vi "Read Meta Data (Serial Clst).vi"(8 "error in":errorcluster, 9 "options":T3={"ignore timeout error"=TRUE, "timeout ms (1000)"=1000}, 11 "connection info in":T1) -> (0 "error out":errorcluster, 1 "meta data":T2[](array[typedef]), 3 "connection info out":T1)   [LabVIEW 2013, in "NI STM.lvlib"]
doc: "This VI reads the meta data information from a remote computer. Use this VI to retrieve the variable names and types that a remote computer exports.\n\nThis VI parses the data and returns a cluster containing the meta data information."
uses:
  NI STM.lvlib
  SubVIs/MetaDataElement.ctl
  Serial Read Options.ctl
  Serial Connection Info.ctl
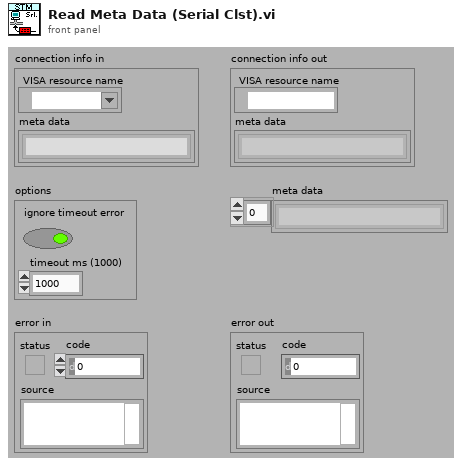
[diagram p1: front panel]
types:
  T1 = typedef "NI STM.lvlib/Serial Connection Info.ctl" = cluster{"VISA resource name":refnum<visa-resource-name>, "meta data":T2[]}
  T2 = typedef "NI STM.lvlib/MetaDataElement.ctl" = string
  T3 = typedef "NI STM.lvlib/Serial Read Options.ctl" = cluster{"ignore timeout error":bool, "timeout ms (1000)":u32}
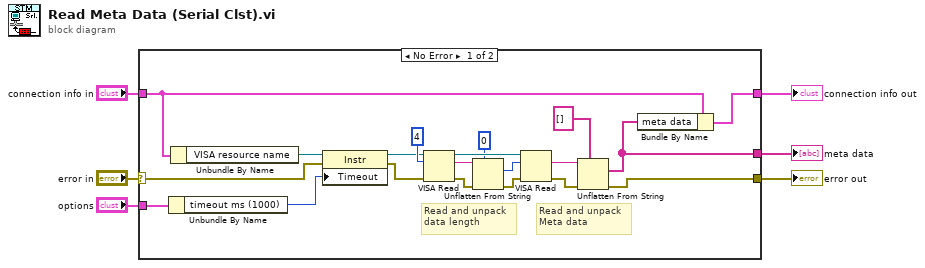
[diagram p0: block diagram]
diagram:
  n1 = case shown="No Error" "error in" {
    selector: "error in" -> [w8 w28]
    tunnel: [w15 _] -> w6
    tunnel: [w26 w28] -> w5
    tunnel: [w14 w27] -> w1
    tunnel: "options" -> [w13 _]
    tunnel: "connection info in" -> [w12 w27]
    frame No Error {
      # "Read and unpack\nMeta data"
      # "Read and unpack\ndata length"
      n2 = Unbundle By Name(w13) -> ("timeout ms (1000)"=w9:u32)
      n3 = Unbundle By Name(w12) -> ("VISA resource name"=w11:refnum<visa-resource-name>)
      n4 = property class="Instr"(reference=w11, error in=w8, "Timeout"=w9) -> (reference out=w10:refnum<visa-resource-name>, error out=w7:errorcluster)
      n5 = VISA Read(VISA resource name=w10, byte count=u32 4 ("bytes to read"), error in (no error)=w7) -> (VISA resource name out=w23:refnum<visa-resource-name>, read buffer=w20:string, error out=w16:errorcluster)  [unwired: 1 out]
      n6 = Unflatten From String(type=u32 0 ("bytes to read"), binary string=w20, error in (no error)=w16) -> (value=w17:u32, error out=w18:errorcluster)  [unwired: 3 out]
      n7 = VISA Read(VISA resource name=w23, byte count=w17, error in (no error)=w18) -> (read buffer=w22:string, error out=w21:errorcluster)  [unwired: 2 out]
      n8 = Unflatten From String(type=T2[] [] ("Meta data"), binary string=w22, error in (no error)=w21) -> (value=w15:T2[], error out=w26:errorcluster)  [unwired: 3 out]
      n9 = Bundle By Name(cluster=w12, "meta data"=w15) -> (w14:T1)
    }
    frame Error {
    }
  }
  "meta data" <- w6
  "error out" <- w5
  "connection info out" <- w1
